vi "testWrite.vi"() -> ()   [LabVIEW 2016]
panel:
  out "error out":errorcluster
  in  "stop":bool
  out "text":string
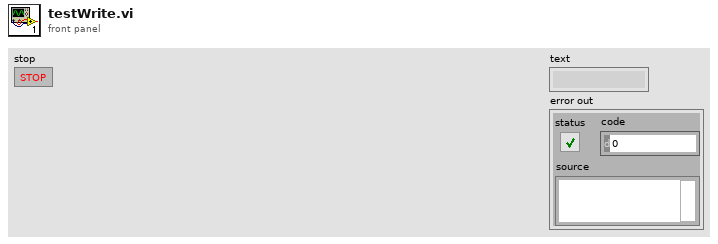
[diagram p1: front panel]
types:
  T1 = enum16{"open", "replace", "create", "open or create", "replace or create", "replace or create with confirmation"}
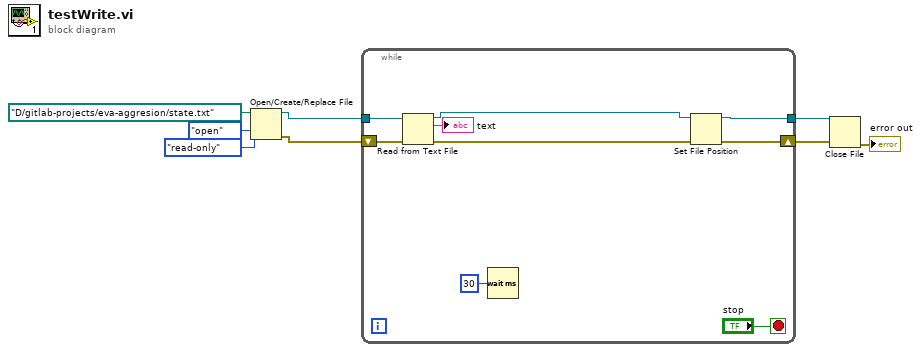
[diagram p0: block diagram]
diagram:
  n1 = Open/Create/Replace File(file path (use dialog)=path "D:/gitlab-projects/eva-aggresion/state.txt", operation (0:open)=T1."open", access (0:read/write)=enum16{"read/write", "read-only", "write-only"}."read-only") -> (refnum out=w5:refnum<file>, error out=w3:errorcluster)  [unwired: 3 in, 1 out]
  n2 = while {
    shift-right: [w10] -> w2
    shift-left: w3 -> [w14]
    tunnel: w5 -> [w17]
    tunnel: [w12] -> w4
    stop <- "stop" stop-if-true
    n3 = Read from Text File(file (use dialog)=w17, error in=w14) -> (refnum out=w13:refnum<file>, text=→"text":string, error out=w11:errorcluster)  [unwired: 2 in, 1 out]
    n4 = Wait (ms)(milliseconds to wait=u32 30) -> ()  [unwired: 1 out]
    n5 = Set File Position(refnum=w13, error in=w11) -> (refnum out=w12:refnum<file>, error out=w10:errorcluster)  [unwired: 2 in]
  }
  n6 = Close File(refnum=w4, error in=w2) -> (error out=→"error out":errorcluster)  [unwired: 1 out]
